vi "poly_notify_name_by_name_single.vi"(8 "error in":errorcluster caption="Error in (no error)", 9 "notifier name":string, 10 "name of caller in (you)":string) -> (0 "error out":errorcluster, 4 "notified?":bool)   [LabVIEW 2015]
uses:
  ref_tools/polys/poly_control_ref_from_name_caller_single.vi
  poly_notify_boolean_notifier_name.vi
  ref_tools/cores/core_ref_tools_eco.vi
  ref_tools/polys/poly_ref_tools_eco_plus.vi
  <vilib>/Utility/error.llb/Clear Errors.vi
  error_tools/toolbox_error_handler.vi
  ref_tools/polys/poly_control_ref_from_name_single.vi
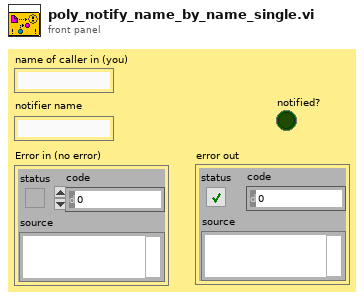
[diagram p1: front panel]
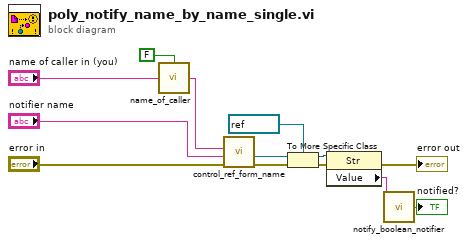
[diagram p0: block diagram]
diagram:
  n1 = call "name_of_caller.vi"("is in inlined vi? (F)"=FALSE, "name of caller in"="name of caller in (you)") -> ("name of caller out"=w6:string)  [unwired: 2 in]
  n2 = call-poly "control_ref_form_name.vi"("error in"="error in", "control name"="notifier name", "name of caller in (your caller)"=w6) -> ("error out"=w9:errorcluster, "control ref"=w13:refnum<vi>)  [unwired: 6 in, 1 out]
  n3 = To More Specific Class(target class=refnum<vi> refnum ("String"), reference=w13, error in=w9) -> (specific class reference=w12:refnum<vi>, error out=w8:errorcluster)
  n4 = property class="Str"(reference=w12, error in=w8) -> (error out=→"error out":errorcluster, "Value"=w2:string)  [unwired: 1 out]
  n5 = call-poly "notify_boolean_notifier.vi"("notifier name"=w2) -> ("notified?"=→"notified?":bool)  [unwired: 8 in]
